vi "SERIALreceive.vi"(2 "timeout ms":u32=4294967295 format="%.0x", 3 "address string":string, 4 "byte count":i32, 9 "error in":errorcluster) -> (0 "read buffer":string, 6 "error out":errorcluster)   [LabVIEW 2013]
doc: "Sends a string to a message based instrument. You must supply the address string of the instrument. A byte count value is required in order to tell the VI how many bytes can be returned by the VI. Select the appropriate read mode to terminate the receive function correctly."
uses:
  <vilib>/Instr/_visa.llb/VISA Configure Serial Port (Instr).vi
panel:
  in  "VISA resource name":refnum<visa-resource-name>
  out "byte count out":i32
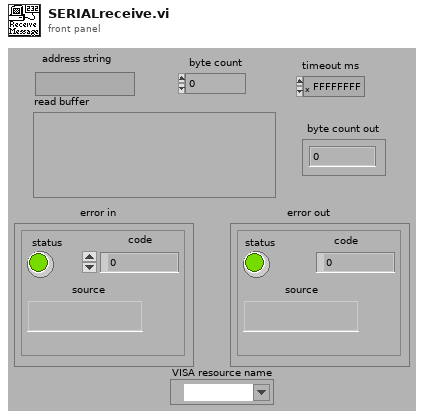
[diagram p1: front panel]
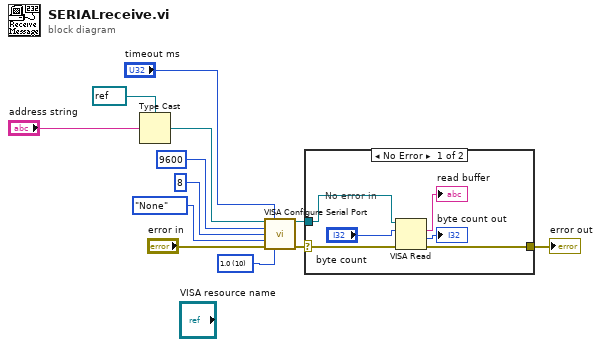
[diagram p0: block diagram]
diagram:
  w3 = u16 10 items=["1.0"=10, "1.5"=15, "2.0"=20] ("stop bits (10: 1 bit)")
  n1 = Type Cast(type=refnum<visa-resource-name> refnum ("VISA resource name"), x="address string") -> (*(type *) &x=w9:refnum<visa-resource-name>)
  n2 = call-poly "VISA Configure Serial Port"("VISA resource name"=w9, "timeout (10sec)"="timeout ms", "baud rate (9600)"=u32 9600, "data bits (8)"=u16 8, "parity (0:none)"=enum16{"None", "Odd", "Even", "Mark", "Space"}."None", "error in (no error)"="error in", "stop bits (10: 1 bit)"=w3) -> ("VISA resource name out"=w8:refnum<visa-resource-name>, "error out"=w2:errorcluster)  [unwired: 7 in]
  n3 = case shown="No Error" w2 {
    selector: w2 -> [w14 w19]
    tunnel: [w15 w19] -> w12
    tunnel: w8 -> [w16 _]
    frame No Error {
      # "No error in"
      n4 = VISA Read(VISA resource name=w16, byte count="byte count", error in (no error)=w14) -> (read buffer=→"read buffer":string, return count=→"byte count out":u32, error out=w15:errorcluster)  [unwired: 1 out]
    }
    frame Error {
      # "Error in"
    }
  }
  "error out" <- w12
